vi "SetCustomCursor.vi"(0 "reference in":refnum<class "LcPictureBox.lvclass">, 2 "CustomCusorIndex":u16, 5 "error in (no error)":errorcluster) -> (14 "reference out":refnum<class "LcPictureBox.lvclass">, 19 "error out":errorcluster)   [LabVIEW 2020, in "LcPictureBox.lvclass"]
uses:
  LcPictureBox.lvclass
  System.Windows.Forms
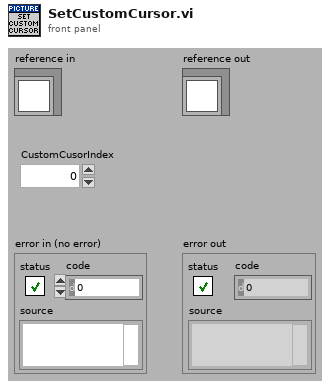
[diagram p1: front panel]
types:
  T1 = typedef "LcPictureBox.lvclass/ObjectAttributes.ctl" = cluster{"PictureBox":refnum<k24>, "ImageSize":cluster{"Width":i32, "Height":i32}, "PenMemory":map{cluster{"Alpha(100%)":dbl, "Color(Black)":u32, "Pen(Width=1, Solid)":T2}, refnum<k24>}, "GraphicsRef":refnum<k24>, "BrushMemory":map{cluster{"Alpha(100%)":dbl, "Color(Black)":u32}, refnum<k24>}, "Images":refnum<k24>[], "ImageIndex":i32, "BgColor(None)":u32, "LoadedImages":map{string, cluster{"ImageOut":refnum<k24>, "ImageSize":cluster{"Width":i32, "Height":i32}}}, "ColorsMemory":map{cluster{"Alpha(100%)":dbl, "Color(Black)":u32}, refnum<k24>}, "CacheSize":i32, "PictureBoxActiveXReference":refnum<vi>, "Scale":dbl, "Offset":cluster{"x":sgl, "y":sgl}, "zoom_center":cluster{"X":i32, "Y":i32}, "ImagesCreated":refnum<k24>[], "CustomCursorImages":map{u16, refnum<k24>}}
  T2 = typedef "LcPictureBox.lvclass/Pen.ctl" = cluster{"Width":u16, "Style":enum32{"Solid", "Dash", "Dot", "DashDot", "DashDotDot"}}
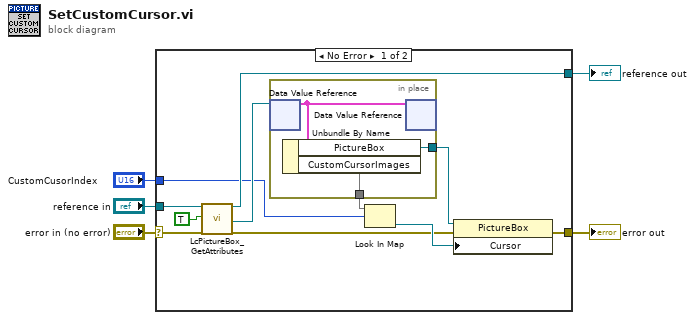
[diagram p0: block diagram]
diagram:
  n1 = case shown="No Error" "error in (no error)" {
    selector: "error in (no error)" -> [w16 w21]
    tunnel: [w13 w21] -> w4
    tunnel: [w14 w20] -> w2
    tunnel: "reference in" -> [w15 w20]
    tunnel: "CustomCusorIndex" -> [w8 _]
    frame No Error {
      n2 = call "LcPictureBox_GetAttributes.vi"("reference in"=w15, "OnlyGetDvrReference(False)"=TRUE, "error in (no error)"=w16) -> ("reference out"=w14:refnum<class "LcPictureBox.lvclass">, "DataRef"=w11:refnum<data-value>, "error out"=w6:errorcluster)  [unwired: 13 in, 1 out]
      n3 = in-place {
        in-place-border: [w19] -> w10
        in-place-border: [w17] -> w9
        n4 = in-place-dvr #1(w11) -> (w18:T1)  [unwired: 1 out]
        n5 = Unbundle By Name(w18) -> ("PictureBox"=w19:refnum<k24>, "CustomCursorImages"=w17:map{u16, refnum<k24>})
        n6 = in-place-dvr #1(w18) -> ()  [unwired: 2 out]
      }
      n7 = Look In Map(map=w9, key=w8) -> (value=w7:refnum<k24>)  [unwired: 1 in, 1 out]
      n8 = property class="PictureBox"(reference=w10, error in=w6, "Cursor"=w7) -> (error out=w13:errorcluster)  [unwired: 1 out]
    }
    frame Error {
    }
  }
  "error out" <- w4
  "reference out" <- w2
